vi "GetAgentsVIs.vi"(3 "error in":errorcluster, 4 "only one Class in Lib?":bool, 5 "Class Path":path) -> (0 "error out":errorcluster, 1 "Agents VI Paths":path[](array[path]), 2 "Agents VI Names":string[](array[string]))   [LabVIEW 2009, in "HGF_VisitorGenerator.lvlib"]
doc: "Get all public member VIs of given Class...these are the interface VIs for the mobile agent system"
uses:
  HGF_VisitorGenerator.lvlib
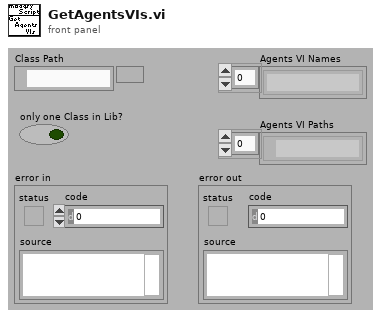
[diagram p1: front panel]
types:
  T1 = enum32{"invalid scope", "public", "private", "protected", "community"}
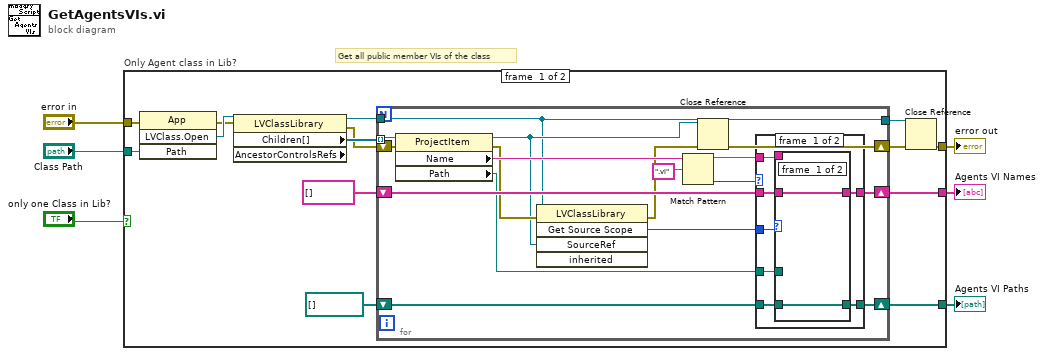
[diagram p0: block diagram]
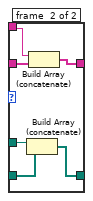
[diagram p2: hidden frame]
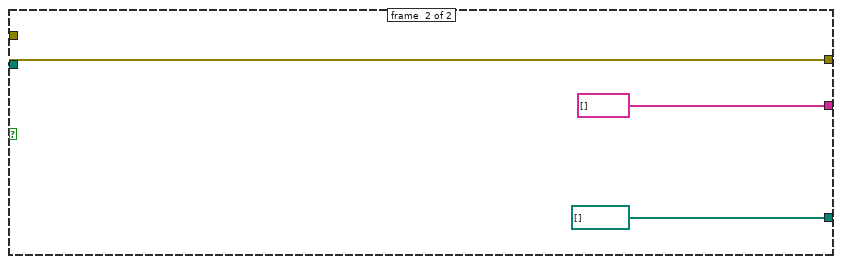
[diagram p4: hidden frame]
diagram:
  # "Get all public member VIs of the class"
  n1 = case "Only Agent class in Lib?" shown="True" "only one Class in Lib?" {
    tunnel: "Class Path" -> [w20 _]
    tunnel: "error in" -> [w18 w55]
    tunnel: [w14 string[] [] ("Array 3")] -> w5
    tunnel: [w13 path[] [] ("Array 2")] -> w6
    tunnel: [w9 w55] -> w1
    frame #0 {
      n2 = invoke class="App" method="LVClass.Open"(error in=w18, "Path"=w20) -> (error out=w17:errorcluster, "LVClass.Open"=w19:refnum<vi>)  [unwired: 2 in, 2 out]
      n3 = property class="LVClassLibrary" props=["Children[]", "AncestorControlsRefs"](reference=w19, error in=w17) -> (reference out=w8:refnum<vi>, error out=w11:errorcluster, "Children[]"=w12:refnum<vi>[])  [unwired: 1 out]
      n4 = for {
        tunnel: w12 -> [w37] mode=indexing
        shift-right: [w30] -> w14
        shift-left: string[] [] ("Array 3") -> [w33]
        shift-right: [w31] -> w13
        shift-left: path[] [] ("Array 2") -> [w32]
        shift-right: [w26] -> w10
        shift-left: w11 -> [w27]
        tunnel: w8 -> [w22]
        tunnel: [w22] -> w7
        n5 = property class="ProjectItem"(reference=w37, error in=w27) -> (reference out=w24:refnum<vi>, error out=w25:errorcluster, "Name"=w36:string, "Path"=w28:path)
        n6 = invoke class="LVClassLibrary" method="Get Source Scope"(reference=w22, error in=w25, "SourceRef"=w24) -> (error out=w23:errorcluster, "GetSourceScope"=w21:T1)  [unwired: 2 in, 3 out]
        n7 = Match Pattern(string=w36, regular expression=".vi") -> (before substring=w29:string, offset past match=w34:i32)  [unwired: 1 in, 2 out]
        n8 = Close Reference(reference=w24, error in (no error)=w23) -> (error out=w26:errorcluster)
        n9 = case shown="0, Default" w34 {
          tunnel: w33 -> [w44 w53]
          tunnel: w32 -> [w41 w54]
          tunnel: [w40 w54] -> w31
          tunnel: [w43 w53] -> w30
          tunnel: w29 -> [w42 _]
          tunnel: w28 -> [w39 _]
          tunnel: w21 -> [w38 _]
          frame #0 {
            n10 = case shown="\"public\"" w38 {
              tunnel: w44 -> [w46 w52]
              tunnel: [w46 w51] -> w43
              tunnel: w42 -> [_ w50]
              tunnel: w41 -> [w45 w49]
              tunnel: [w45 w48] -> w40
              tunnel: w39 -> [_ w47]
              frame #0 {
              }
              frame #1 {
                n11 = Build Array (concatenate)(w47, w49) -> (w48:path[])
                n12 = Build Array (concatenate)(w50, w52) -> (w51:string[])
              }
            }
          }
          frame #1 {
          }
        }
      }
      n13 = Close Reference(reference=w7, error in (no error)=w10) -> (error out=w9:errorcluster)
    }
    frame #1 {
    }
  }
  "Agents VI Paths" <- w6
  "Agents VI Names" <- w5
  "error out" <- w1
